vi "Update Min Max.vi"(0 "TDMS In":refnum<k34>, 5 "Group":string, 7 "Channels":string[](array[string]), 9 "Value/Channel":sgl[][](array[numeric]), 11 "Error In":errorcluster) -> (4 "TDMS Out":refnum<k34>, 15 "Error Out":errorcluster)   [LabVIEW 2015, in "Teaching File.lvlib"]
doc: "Check the values and compare them to min and max properties stored for each channel. Update the properties with correct min and max values."
uses:
  Teaching File.lvlib
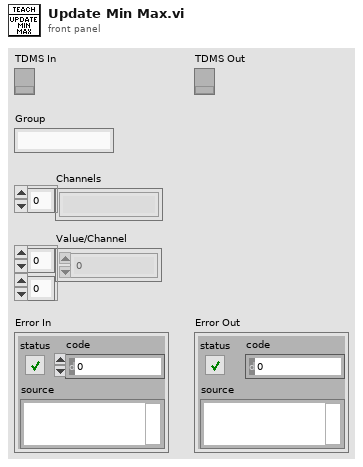
[diagram p1: front panel]
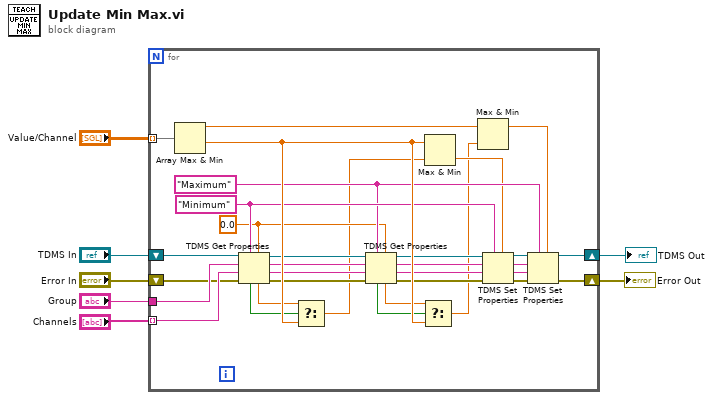
[diagram p0: block diagram]
diagram:
  n1 = for {
    tunnel: "Value/Channel" -> [w33] mode=indexing
    tunnel: "Channels" -> [w39] mode=indexing
    tunnel: "Group" -> [w36]
    shift-right: [w38] -> w5
    shift-left: "TDMS In" -> [w35]
    shift-right: [w37] -> w4
    shift-left: "Error In" -> [w34]
    w14 = sgl 0.0
    w17 = "Maximum" ("group name in")
    w18 = "Minimum" ("group name in")
    n2 = Array Max & Min(array=w33) -> (max value=w31:sgl, min value=w32:sgl)  [unwired: 2 out]
    n3 = TDMS Get Properties(5:w14, 7:w18, 8:w34, 9:w39, 10:w36, 11:w35) -> (0:w22:errorcluster, 1:w20:string, 2:w19:string, 3:w21:refnum<k34>, 4:w10:sgl, 6:w9:bool)
    n4 = Select(t=w10, s=w9, f=w32) -> (s? t:f=w8:sgl)
    n5 = TDMS Get Properties(5:w14, 7:w17, 8:w22, 9:w20, 10:w19, 11:w21) -> (0:w26:errorcluster, 1:w23:string, 2:w24:string, 3:w25:refnum<k34>, 4:w12:sgl, 6:w13:bool)
    n6 = Select(t=w12, s=w13, f=w32) -> (s? t:f=w11:sgl)
    n7 = Max & Min(x=w32, y=w8) -> (min(x,y)=w16:sgl)  [unwired: 1 out]
    n8 = Max & Min(x=w31, y=w11) -> (max(x,y)=w15:sgl)  [unwired: 1 out]
    n9 = TDMS Set Properties(5:w16, 7:w18, 8:w26, 9:w23, 10:w24, 11:w25) -> (0:w30:errorcluster, 1:w28:string, 2:w27:string, 3:w29:refnum<k34>)
    n10 = TDMS Set Properties(5:w15, 7:w17, 8:w30, 9:w28, 10:w27, 11:w29) -> (0:w37:errorcluster, 3:w38:refnum<k34>)  [unwired: 2 out]
  }
  "TDMS Out" <- w5
  "Error Out" <- w4
